vi "ShiftRegisterForWhile.vi"() -> ()   [LabVIEW 2020]
panel:
  out "Numeric":dbl
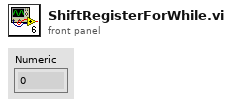
[diagram p1: front panel]
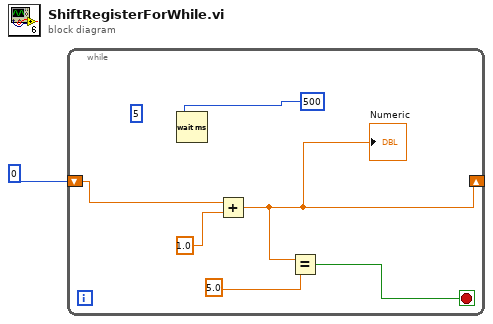
[diagram p0: block diagram]
diagram:
  n1 = while {
    shift-right: [w5] -> _
    shift-left: 0 -> [w6]
    stop <- w3 stop-if-true
    (unwired) 5
    n2 = Wait (ms)(milliseconds to wait=u32 500) -> ()  [unwired: 1 out]
    n3 = Add(x=w6, y=1.0) -> (x+y=w5:dbl)
    "Numeric" <- w5
    n4 = Equal?(x=w5, y=5.0) -> (x = y?=w3:bool)
  }
